vi "FABR-Init AvsF Plot.vi"(0 "Graph":refnum<vi>, 2 "FreqAxisLabel":refnum<vi>, 5 "Legend":refnum<vi>, 7 "Freq":dbl[](array[numeric]), 9 "Level":dbl[](array[numeric]), 11 "error in (no error)":errorcluster) -> (15 "error out":errorcluster)   [LabVIEW 2020]
uses:
  epl-vi-lib/Utility VIs/Math VIs/LinSpace (x0-dx-npts).vi
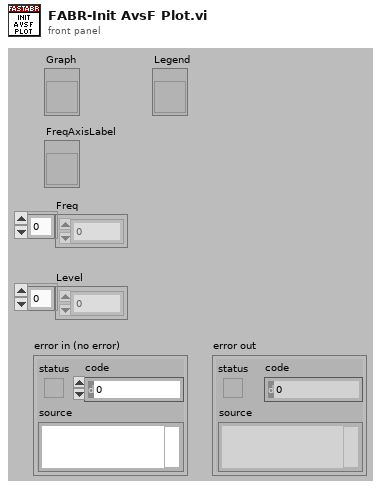
[diagram p1: front panel]
types:
  T1 = enum16{"User", "Prism", "Kelly", "Dark2", "Sequential", "Hue"}
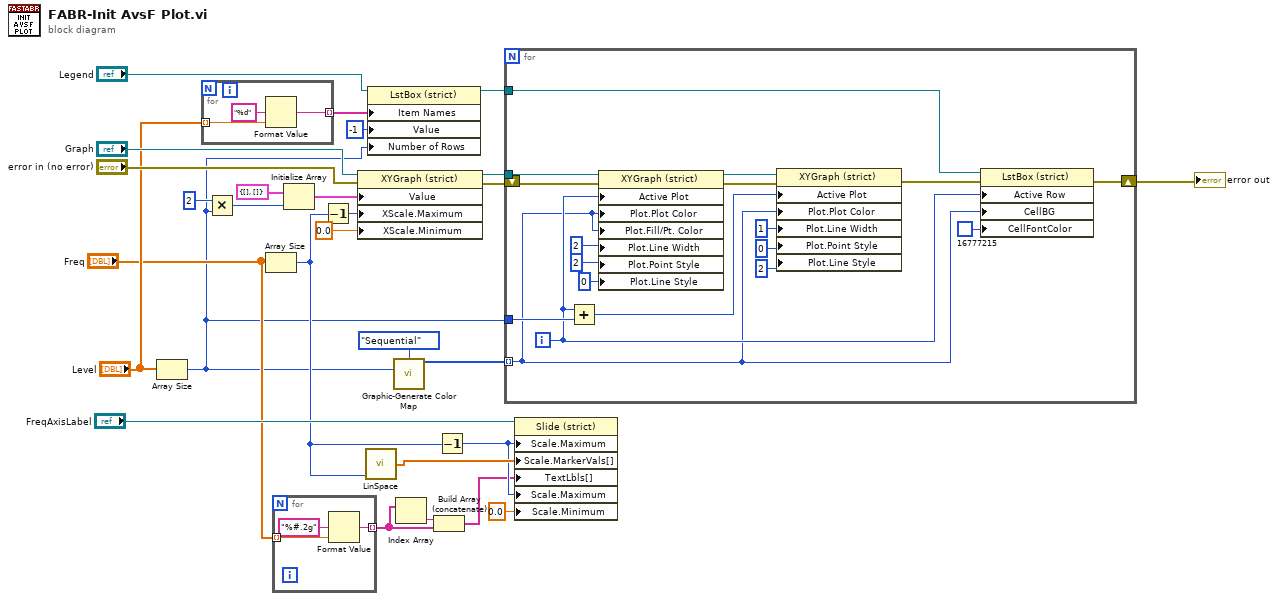
[diagram p0: block diagram]
diagram:
  n1 = Array Size(array="Level") -> (size(s)=w1:i32)
  n2 = for {
    tunnel: "Level" -> [w31] mode=indexing
    tunnel: [w29] -> w16 mode=indexing
    n3 = Format Value(format string="%d", value (0)=w31) -> (output string=w29:string)  [unwired: 1 in]
  }
  n4 = Multiply(x=2, y=w1) -> (x*y=w23:i32)
  n5 = Array Size(array="Freq") -> (size(s)=w8:i32)
  n6 = for {
    tunnel: "Freq" -> [w34] mode=indexing
    tunnel: [w32] -> w3 mode=indexing
    n7 = Format Value(format string="%#.2g", value (0)=w34) -> (output string=w32:string)  [unwired: 1 in]
  }
  n8 = Initialize Array(cluster{dbl[], dbl[]} {[], []}, w23) -> (w22:cluster{dbl[], dbl[]}[])
  n9 = Decrement(x=w8) -> (x-1=w5:i32)
  n10 = property class="XYGraph (strict)"(reference="Graph", error in="error in (no error)", "Value"=w22, "XScale.Maximum"=w5, "XScale.Minimum"=0.0 ("X Scale.Range:Maximum")) -> (reference out=w21:refnum<vi>, error out=w20:errorcluster)
  n11 = call-poly "LinSpace.vi"("npts"=w8) -> ("Array"=w11:dbl[])  [unwired: 3 in, 1 out]
  n12 = property class="LstBox (strict)"(reference="Legend", "Item Names"=w16, "Value"=-1 ("Focus Row"), "Number of Rows"=w1) -> (reference out=w15:refnum<vi>)  [unwired: 1 in, 1 out]
  n13 = call "Graphic-Generate Color Map.vi"("Map"=T1."Sequential", "Size"=w1) -> ("Colors"=w19:u32[])  [unwired: 13 in]
  n14 = Index Array(array=w3) -> (element=w2:string)  [unwired: 1 in]
  n15 = Build Array (concatenate)(w2, w3) -> (w4:string[])
  n16 = Decrement(x=w8) -> (x-1=w6:i32)
  n17 = for {
    tunnel: w21 -> [w52]
    tunnel: w19 -> [w36] mode=indexing
    tunnel: w1 -> [w46]
    shift-right: [w38] -> w18
    shift-left: w20 -> [w51]
    tunnel: w15 -> [w40]
    i -> [w37]
    n18 = Add(x=w37, y=w46) -> (x+y=w45:i32)
    n19 = property class="XYGraph (strict)"(reference=w52, error in=w51, "Active Plot"=w37, "Plot.Plot Color"=w36, "Plot.Fill/Pt. Color"=w36, "Plot.Line Width"=u8 2, "Plot.Point Style"=u8 2, "Plot.Line Style"=u8 0) -> (reference out=w48:refnum<vi>, error out=w47:errorcluster)
    n20 = property class="XYGraph (strict)"(reference=w48, error in=w47, "Active Plot"=w45, "Plot.Plot Color"=w36, "Plot.Line Width"=u8 1, "Plot.Point Style"=u8 0, "Plot.Line Style"=u8 2) -> (error out=w39:errorcluster)  [unwired: 1 out]
    n21 = property class="LstBox (strict)"(reference=w40, error in=w39, "Active Row"=w37, "CellBG"=w36, "CellFontColor"=u32 16777215) -> (error out=w38:errorcluster)  [unwired: 1 out]
  }
  "error out" <- w18
  n22 = property class="Slide (strict)"(reference="FreqAxisLabel", "Scale.Maximum"=w6, "Scale.MarkerVals[]"=w11, "TextLbls[]"=w4, "Scale.Maximum"=w6, "Scale.Minimum"=0.0 ("Scale.Range:Minimum")) -> ()  [unwired: 1 in, 2 out]
